vi "Validate Fixed Header.vi"(8 "error in (no error)":errorcluster, 11 "PUBCOMP in":refnum<class "PUBCOMP.lvclass">) -> (0 "error out":errorcluster, 1 "Valid":bool, 3 "PUBCOMP out":refnum<class "PUBCOMP.lvclass">)   [LabVIEW 2013, in "MQTT_Control_Packets.lvlib" / "PUBCOMP.lvclass"]
uses:
  PUBCOMP.lvclass
  ControlPacket/ControlPacket.lvclass/ControlPacket.ctl
  ControlPacket/ControlPacket.lvclass
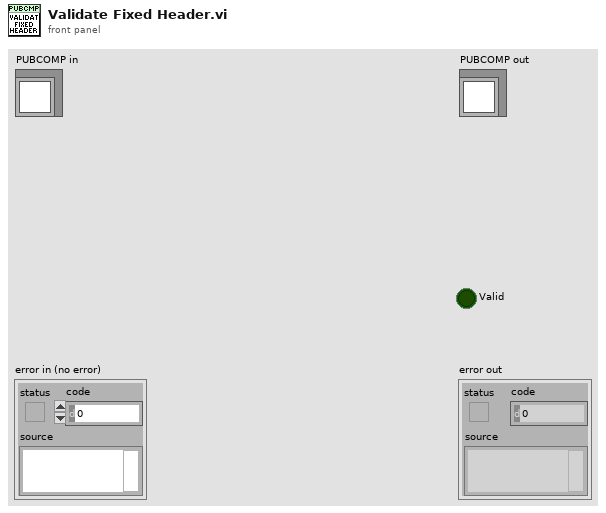
[diagram p1: front panel]
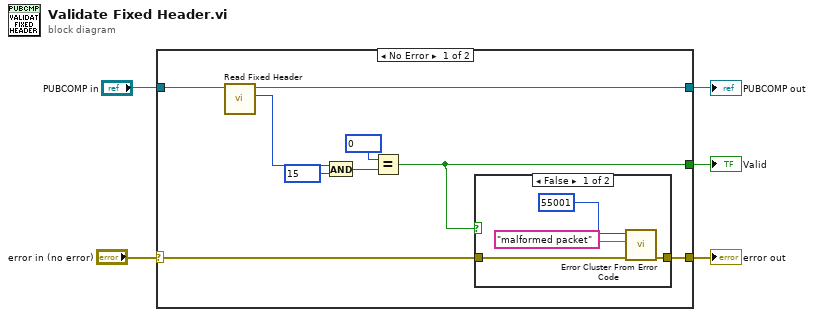
[diagram p0: block diagram]
diagram:
  n1 = case shown="No Error" "error in (no error)" {
    selector: "error in (no error)" -> [w12 w21]
    tunnel: [w11 w21] -> w3
    tunnel: [w6 _] -> w2
    tunnel: [w7 w20] -> w1
    tunnel: "PUBCOMP in" -> [w13 w20]
    frame No Error {
      n2 = call "Read Fixed Header.vi"("ControlPacket in"=w13) -> ("Fixed Header"=w10:u8, "ControlPacket out"=w7:refnum<class "PUBCOMP.lvclass">)  [unwired: 9 in]
      n3 = And(x=w10, y=u8 15) -> (x .and. y?=w9:u8)
      n4 = Equal?(x=u8 0 ("y"), y=w9) -> (x = y?=w6:bool)
      n5 = case shown="False" w6 {
        tunnel: [w16 w19] -> w11
        tunnel: w12 -> [w15 w19]
        frame False {
          n6 = call <vilib>:"Error Cluster From Error Code.vi"("error in (no error)"=w15, "error message (\"\")"="malformed packet" ("error message (\"\")"), "error code (0)"=55001) -> ("error out"=w16:errorcluster)  [unwired: 6 in]
        }
        frame True {
        }
      }
    }
    frame Error {
    }
  }
  "Valid" <- w2
  "error out" <- w3
  "PUBCOMP out" <- w1
